vi "Two LightField Instances.vi"() -> ()   [LabVIEW 2013]
uses:
  lightfield-automation-labview/LightField Automation.lvclass
panel:
  in  "ExperimentName 2":string
  in  "ExperimentName":string
  in  "stop":bool
  in  "Exposure Time (s) 2":dbl(knob)=92.509 step=0.001 scale=0.0..1000.0
  in  "Exposure Time (s)":dbl(knob)=430.129 step=0.001 scale=0.0..1000.0
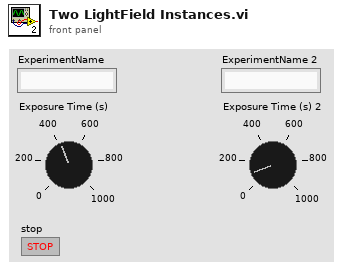
[diagram p1: front panel]
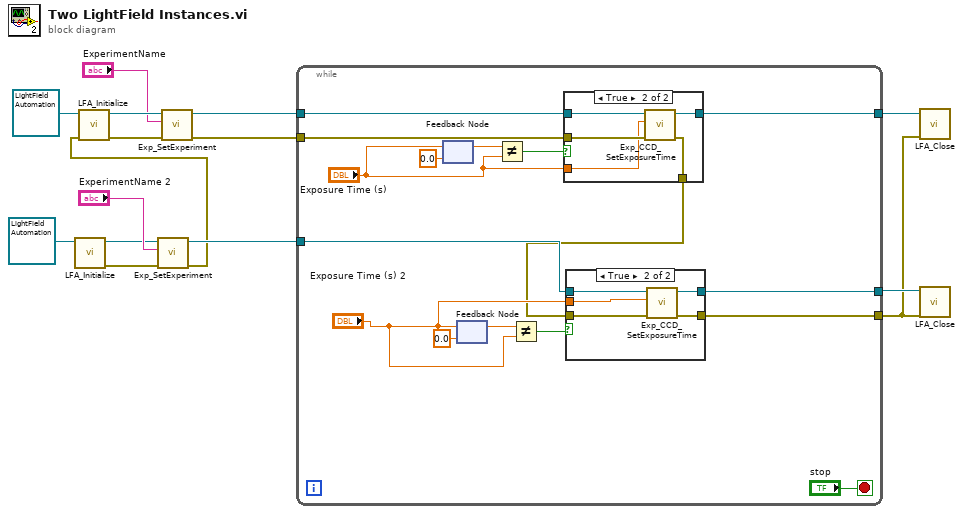
[diagram p0: block diagram]
diagram:
  n1 = call "LFA_Initialize.vi"("LightField Automation in"=refnum<class "LightField Automation.lvclass"> refnum ("LightField Automation.lvclass")) -> ("error out"=w9:errorcluster, "LightField Automation out"=w8:refnum<class "LightField Automation.lvclass">)  [unwired: 9 in]
  n2 = call "Exp_SetExperiment.vi"("error in (no error)"=w9, "ExperimentName"="ExperimentName 2", "LightField Automation in"=w8) -> ("error out"=w5:errorcluster, "LightField Automation out"=w6:refnum<class "LightField Automation.lvclass">)  [unwired: 7 in]
  n3 = call "LFA_Initialize.vi"("error in (no error)"=w5, "LightField Automation in"=refnum<class "LightField Automation.lvclass"> refnum ("LightField Automation.lvclass")) -> ("error out"=w13:errorcluster, "LightField Automation out"=w14:refnum<class "LightField Automation.lvclass">)  [unwired: 8 in]
  n4 = call "Exp_SetExperiment.vi"("error in (no error)"=w13, "ExperimentName"="ExperimentName", "LightField Automation in"=w14) -> ("error out"=w4:errorcluster, "LightField Automation out"=w11:refnum<class "LightField Automation.lvclass">)  [unwired: 7 in]
  n5 = while {
    tunnel: w6 -> [w22]
    tunnel: w11 -> [w28]
    tunnel: w4 -> [w27]
    tunnel: [w20] -> w2
    tunnel: [w19] -> w3
    tunnel: [w18] -> w1
    stop <- "stop" stop-if-true
    n6 = feedback-in #1("Exposure Time (s)") -> ()
    n7 = feedback #1(0.0 ("Exposure Time (s)")) -> (w31:dbl)
    n8 = feedback #2(0.0 ("Exposure Time (s)")) -> (w25:dbl)
    n9 = feedback-in #2("Exposure Time (s) 2") -> ()
    n10 = Not Equal?(x=w31, y="Exposure Time (s)") -> (x != y?=w29:bool)
    n11 = Not Equal?(x=w25, y="Exposure Time (s) 2") -> (x != y?=w24:bool)
    n12 = case shown="True" w29 {
      tunnel: w28 -> [w39 w45]
      tunnel: w27 -> [w40 w44]
      tunnel: [w40 w43] -> w21
      tunnel: [w39 w42] -> w20
      tunnel: "Exposure Time (s)" -> [_ w41]
      frame False {
      }
      frame True {
        n13 = call "Exp_CCD_SetExposureTime.vi"("error in (no error)"=w44, "Exposure Time (s)"=w41, "LightField Automation in"=w45) -> ("error out"=w43:errorcluster, "LightField Automation out"=w42:refnum<class "LightField Automation.lvclass">)  [unwired: 7 in]
      }
    }
    n14 = case shown="True" w24 {
      tunnel: w22 -> [w33 w38]
      tunnel: w21 -> [w32 w37]
      tunnel: "Exposure Time (s) 2" -> [_ w36]
      tunnel: [w33 w35] -> w19
      tunnel: [w32 w34] -> w18
      frame False {
      }
      frame True {
        n15 = call "Exp_CCD_SetExposureTime.vi"("error in (no error)"=w37, "Exposure Time (s)"=w36, "LightField Automation in"=w38) -> ("error out"=w34:errorcluster, "LightField Automation out"=w35:refnum<class "LightField Automation.lvclass">)  [unwired: 7 in]
      }
    }
  }
  n16 = call "LFA_Close.vi"("error in (no error)"=w1, "LightField Automation in"=w2) -> ()  [unwired: 8 in, 2 out]
  n17 = call "LFA_Close.vi"("error in (no error)"=w1, "LightField Automation in"=w3) -> ()  [unwired: 8 in, 2 out]
